vi "FGV - License Info.vi"(6 "FGV States":enum16{"Read", "Write"}(ring), 8 "Error In":errorcluster, 11 "License Info  In":T1={"Expired Time"="", "Computer ID"="", "Product Name"="", "Period"=0, "Activated Time"="", "License Level"=enum."Level 1", "License Type"=enum."Trial", "Log Time"=""}) -> (0 "Error Out":errorcluster, 3 "License Info":T1={"Expired Time"="", "Computer ID"="", "Product Name"="", "Period"=0, "Activated Time"="", "License Level"=enum."Level 1", "License Type"=enum."Trial", "Log Time"=""})   [LabVIEW 2020]
uses:
  Control/License File Parameter.ctl
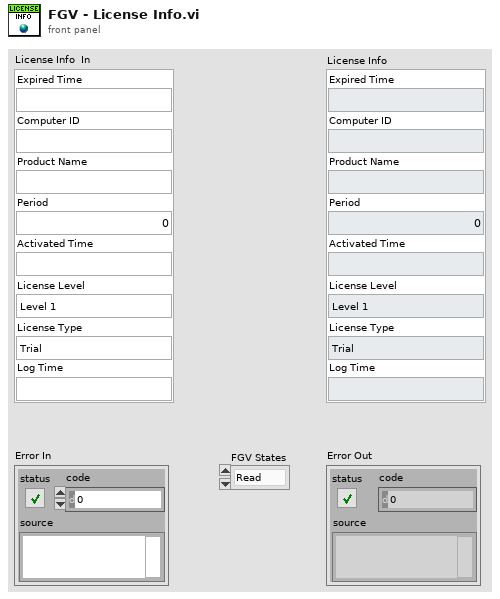
[diagram p1: front panel]
types:
  T1 = typedef "License File Parameter.ctl" = cluster{"Expired Time":string, "Computer ID":string, "Product Name":string, "Period":i16, "Activated Time":string, "License Level":enum16{"Level 1", "Level 2", "Level 3", "Level 4", "Level 5"}, "License Type":enum16{"Free", "Trial", "Subscription", "Perpetual"}, "Log Time":string}
  T2 = cluster{"Computer ID":string, "Validity":string, "Level":string}
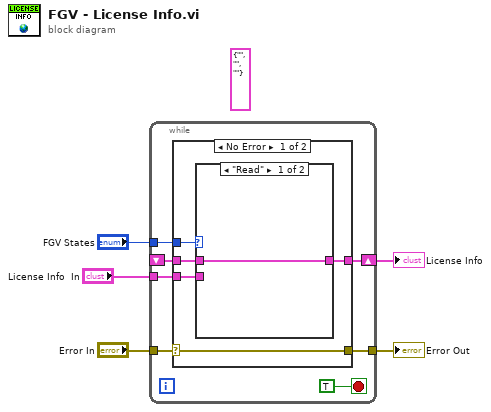
[diagram p0: block diagram]
diagram:
  (unwired) T2 {"Computer ID"="", "Validity"="", "Level"=""} ("License Info In")
  n1 = while {
    tunnel: "Error In" -> [w12]
    tunnel: [w11] -> w4
    tunnel: "FGV States" -> [w9]
    tunnel: "License Info  In" -> [w8]
    shift-right: [w7] -> w1
    shift-left: _ -> [w6]
    stop <- TRUE stop-if-true
    n2 = case shown="No Error" w12 {
      selector: w12 -> [w17 w21]
      tunnel: [w17 w21] -> w11
      tunnel: w9 -> [w16 _]
      tunnel: w8 -> [w15 _]
      tunnel: [w14 w20] -> w7
      tunnel: w6 -> [w13 w20]
      frame No Error {
        n3 = case shown="\"Read\"" w16 {
          tunnel: w15 -> [_ w19]
          tunnel: [w18 w19] -> w14
          tunnel: w13 -> [w18 _]
          frame "Read" {
          }
          frame "Write" {
          }
        }
      }
      frame Error {
      }
    }
  }
  "Error Out" <- w4
  "License Info" <- w1
